vi "m1m3_logEvent_ForceActuatorForceWarning.vi"(8 "error in (no error)":errorcluster, 11 "logevent_ForceActuatorForceWarning_Ctl":T1) -> (0 "error out":errorcluster, 2 "function return":i32, 3 "logevent_ForceActuatorForceWarning_Ctl out":T1)   [LabVIEW 2016, in "SALLV_m1m3.lvlib"]
doc: "int m1m3_shm_logEvent_ForceActuatorForceWarningLV(m1m3_logevent_ForceActuatorForceWarningLV *logevent_ForceActuatorForceWarning_Ctl );"
uses:
  SALLV_m1m3.lvlib
  DataTypes/logevent_ForceActuatorForceWarning.ctl
  SALLV_m1m3.so
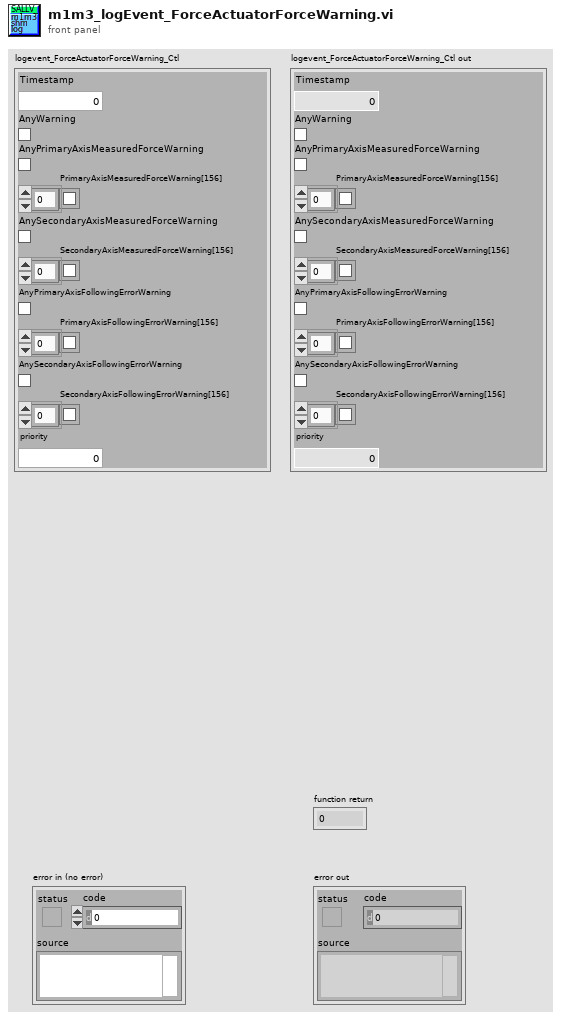
[diagram p1: front panel]
types:
  T1 = typedef "SALLV_m1m3.lvlib/logevent_ForceActuatorForceWarning.ctl" = cluster{"Timestamp":dbl, "AnyWarning":bool, "AnyPrimaryAxisMeasuredForceWarning":bool, "PrimaryAxisMeasuredForceWarning[156]":bool[], "AnySecondaryAxisMeasuredForceWarning":bool, "SecondaryAxisMeasuredForceWarning[156]":bool[], "AnyPrimaryAxisFollowingErrorWarning":bool, "PrimaryAxisFollowingErrorWarning[156]":bool[], "AnySecondaryAxisFollowingErrorWarning":bool, "SecondaryAxisFollowingErrorWarning[156]":bool[], "priority":i32}
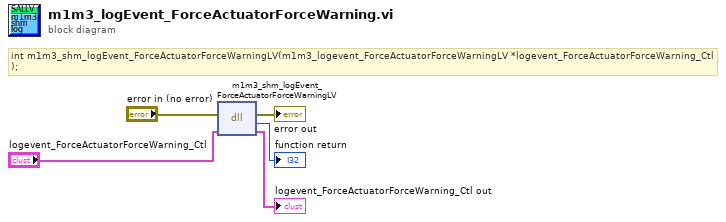
[diagram p0: block diagram]
diagram:
  # "int m1m3_shm_logEvent_ForceActuatorForceWarningLV(m1m3_logevent_ForceActuatorForceWarningLV *logevent_ForceActuatorForceWarning_Ctl );"
  n1 = dll-call lib="opt/CODE/SALLV_m1m3/SALLV_m1m3.*" fn="m1m3_shm_logEvent_ForceActuatorForceWarningLV"(error in="error in (no error)", "logevent_ForceActuatorForceWarning_Ctl"="logevent_ForceActuatorForceWarning_Ctl") -> (error out=→"error out":errorcluster, →"function return":i32, "logevent_ForceActuatorForceWarning_Ctl"=→"logevent_ForceActuatorForceWarning_Ctl out":T1)  [unwired: 2 in, 1 out]
